vi "Test gRPC cRIO XNET Read Raw Frame.vi"(11 "Test Case In":refnum<class "Test Communicator gRPC.lvclass">) -> (0 "error out":errorcluster, 3 "Test Case Out":refnum<class "Test Communicator gRPC.lvclass">)   [LabVIEW 2025, in "Test Communicator gRPC.lvclass"]
uses:
  Test Communicator gRPC.lvclass
  Test Communicator gRPC.lvclass/Test Communicator gRPC.ctl
  Source/Configure Strategies/gRPC XNET Read Raw CAN Frame Strategy/gRPC XNET Read Raw CAN Frame Strategy.lvclass
  D:/git/HAL/Source/Interfaces/IConfigure/IConfigure.lvclass
  D:/git/HAL/Source/Interfaces/IClose/IClose.lvclass
  D:/git/HAL/Source/Interfaces/IInitialize/IInitialize.lvclass
  D:/git/HAL/HAL-Devices/Source/Configure Strategies/gRPC XNET Read Raw CAN Frame Strategy/gRPC XNET Read Raw CAN Frame Strategy.lvclass
  D:/git/HAL/Source/Interfaces/ICommunicate/ICommunicate.lvclass
  D:/git/HAL/Source/Interfaces/IRunnable/IRunnable.lvclass
  C:/Program Files/National Instruments/LabVIEW 2025/vi.lib/Astemes/LUnit/Test Case.lvclass
  C:/Program Files/National Instruments/LabVIEW 2025/vi.lib/Astemes/LUnit/LUnit Runnable.lvclass
  D:/git/HAL/HAL-Devices/Tests/New folder/Test Communicator gRPC.lvclass
  <vilib>/Astemes/LUnit/Test Case.lvclass
  Source/Interfaces/IMessage/IMessage.lvclass
  Source/Communicator/Communicator.lvclass
panel:
  out "Timestamp":timestamp
  out "Data":u8[](array[numeric]) format="%.0x"
  out "Identifier":string
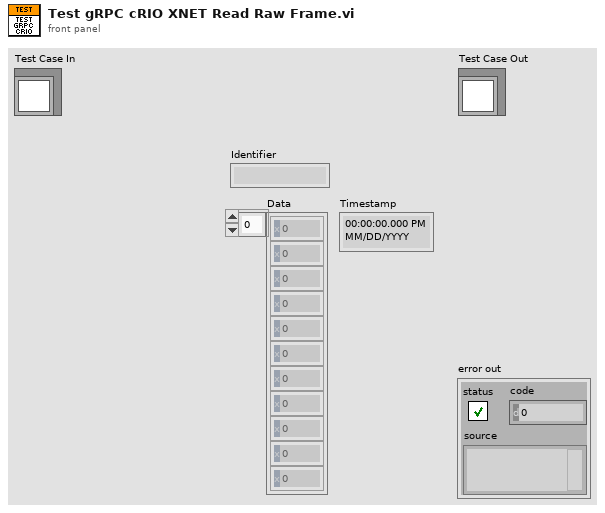
[diagram p1: front panel]
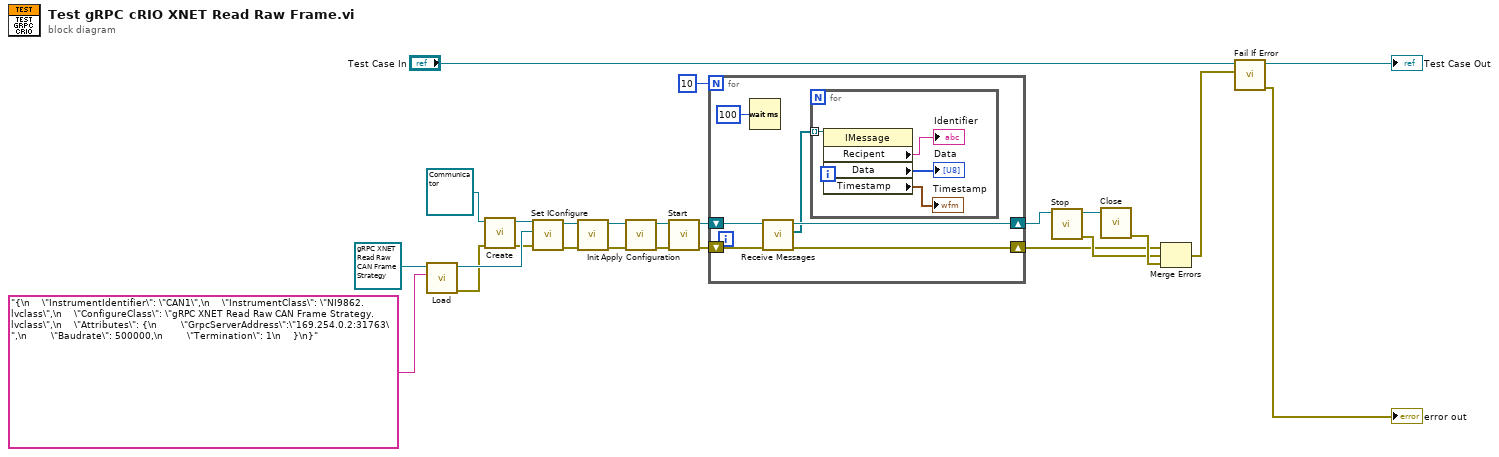
[diagram p0: block diagram]
diagram:
  n1 = call-dynamic "Load.vi"("Source"="{\n    \"InstrumentIdentifier\": \"CAN1\",\n    \"InstrumentClass\": \"NI9862.lvclass\",\n    \"ConfigureClass\": \"gRPC XNET Read Raw CAN Frame Strategy.lvclass\",\n    \"Attributes\": {\n        \"GrpcServerAddress\":\"169.254.0.2:31763\",\n        \"Baudrate\": 500000,\n        \"Termination\": 1\n    }\n}", "gRPC XNET Read Raw CAN Frame Strategy in"=refnum<class "gRPC XNET Read Raw CAN Frame Strategy.lvclass"> refnum ("IConfigure")) -> ("error out"=w4:errorcluster, "gRPC XNET Read Raw CAN Frame Strategy out"=w22:refnum<class "gRPC XNET Read Raw CAN Frame Strategy.lvclass">)  [unwired: 8 in]
  n2 = call-dynamic "Create.vi"("Error In"=w4, "reference in"=refnum<class "Communicator.lvclass"> refnum ("Communicator in")) -> ("Error Out"=w1:errorcluster, "reference out"=w2:refnum<class "Communicator.lvclass">)  [unwired: 8 in]
  n3 = call-dynamic "Set IConfigure.vi"("Error In"=w1, "IConfigure"=w22, "Communicator in"=w2) -> ("Error Out"=w20:errorcluster, "Communicator out"=w19:refnum<class "Communicator.lvclass">)  [unwired: 7 in]
  n4 = call-dynamic "Init.vi"("Error In"=w20, "Communicator in"=w19) -> ("Error Out"=w18:errorcluster, "Communicator out"=w17:refnum<class "Communicator.lvclass">)  [unwired: 8 in]
  n5 = call-dynamic "Apply Configuration.vi"("Error In"=w18, "Communicator in"=w17) -> ("Error Out"=w10:errorcluster, "Communicator out"=w11:refnum<class "Communicator.lvclass">)  [unwired: 8 in]
  n6 = call-dynamic "Start.vi"("Error In"=w10, "Communicator in"=w11) -> ("Error Out"=w14:errorcluster, "Communicator out"=w15:refnum<class "Communicator.lvclass">)  [unwired: 8 in]
  n7 = for {
    N: 10 -> [_]
    shift-right: [w29] -> w13
    shift-left: w15 -> [w31]
    shift-right: [w28] -> w6
    shift-left: w14 -> [w30]
    n8 = Wait (ms)(milliseconds to wait=u32 100) -> ()  [unwired: 1 out]
    n9 = call-dynamic "Receive Messages.vi"("Error In"=w30, "Communicator in"=w31) -> ("Error Out"=w28:errorcluster, "Messages"=w27:refnum<class "IMessage.lvclass">[], "Communicator out"=w29:refnum<class "Communicator.lvclass">)  [unwired: 7 in]
    n10 = for {
      tunnel: w27 -> [w35] mode=indexing
      n11 = property class="IMessage"(reference=w35) -> ("Recipent"=→"Identifier":string, "Data"=→"Data":u8[], "Timestamp"=→"Timestamp":timestamp)  [unwired: 1 in, 2 out]
    }
  }
  n12 = call-dynamic "Stop.vi"("Communicator in"=w13) -> ("Error Out"=w7:errorcluster, "Communicator out"=w12:refnum<class "Communicator.lvclass">)  [unwired: 9 in]
  n13 = call-dynamic "Close.vi"("Communicator in"=w12) -> ("Error Out"=w9:errorcluster)  [unwired: 9 in, 1 out]
  n14 = Merge Errors(w6, w7, w9) -> (w8:errorcluster)
  n15 = call <vilib>:"Fail If Error.vi"("Assert error"=w8, "LUnit Test Case In"="Test Case In") -> ("error out"=→"error out":errorcluster, "LUnit Test Case Out"=→"Test Case Out":refnum<class "Test Communicator gRPC.lvclass">)  [unwired: 8 in]
